vi "WriteResolverParameters.vi"(8 "error in (no error)":errorcluster, 9 "UserValues":dbl[](array[numeric]), 10 "Resolver Parameters in":T1[](array[typedef]), 11 "FPGA Session":u32) -> (0 "error out":errorcluster, 2 "Resolver Parameters out":T1[](array[typedef]), 3 "FPGA Session Out":u32)   [LabVIEW 2011, in "Sensor Simulation Custom Device.lvlib"]
uses:
  Sensor Simulation Custom Device.lvlib
  TypeDefs/Resolver Parameters.ctl
  <userlib>/_FPGA Interface Advanced Tools/FPGA Interface Wrapper/NiFPGA Write - I32.vi
  <vilib>/Utility/error.llb/Error Cluster From Error Code.vi
  <userlib>/_FPGA Interface Advanced Tools/FPGA Interface Wrapper/FPGA Interface Wrapper.lvlib
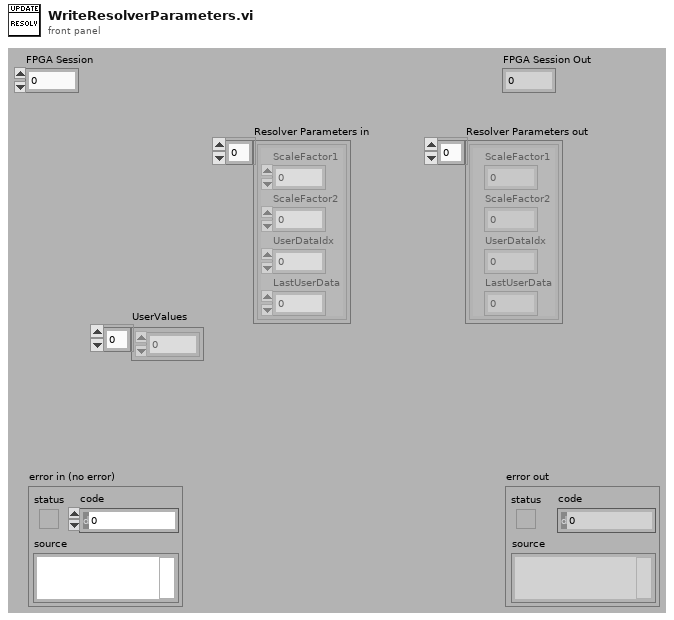
[diagram p1: front panel]
types:
  T1 = typedef "Sensor Simulation Custom Device.lvlib/Resolver Parameters.ctl" = cluster{"ScaleFactor1":u32, "ScaleFactor2":u32, "UserDataIdx":i32, "LastUserData":dbl}
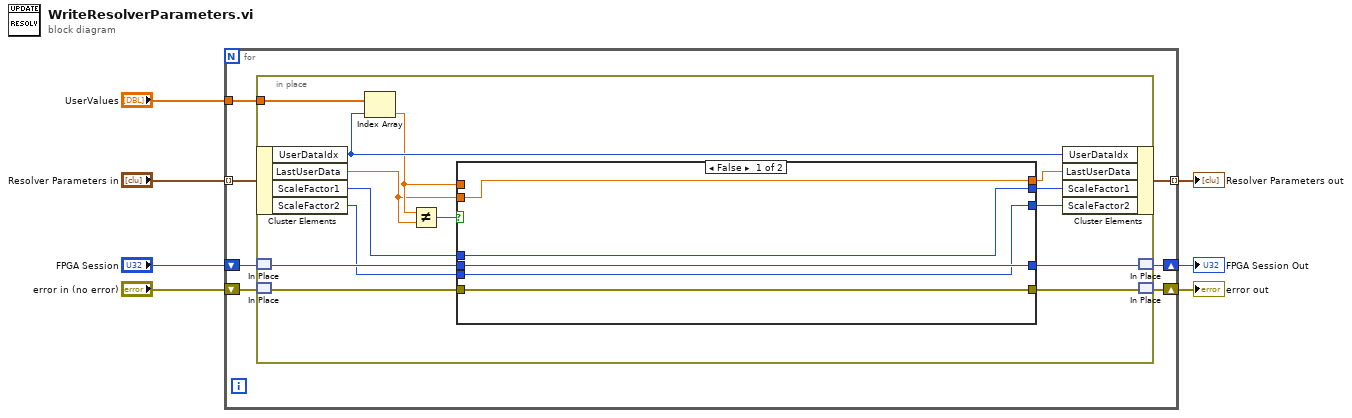
[diagram p0: block diagram]
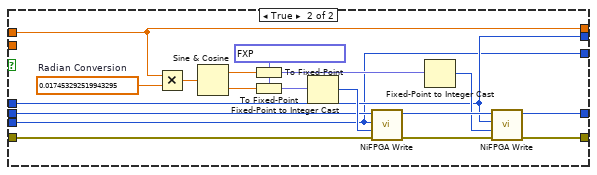
[diagram p2: hidden frame]
diagram:
  n1 = for {
    shift-right: [w11] -> w6
    shift-left: "error in (no error)" -> [w12]
    shift-right: [w10] -> w5
    shift-left: "FPGA Session" -> [w13]
    tunnel: "UserValues" -> [w14]
    tunnel: "Resolver Parameters in" -> [w9] mode=indexing
    tunnel: [w8] -> w1 mode=indexing
    n2 = in-place {
      in-place-border: w14 -> [w28]
      n3 = in-place-cluster #1(w9) -> ("UserDataIdx"=w23:i32, "LastUserData"=w19:dbl, "ScaleFactor1"=w18:u32, "ScaleFactor2"=w17:u32)
      n4 = in-place-match #2(w13) -> (w26:u32)
      n5 = in-place-match #3(w12) -> (w27:errorcluster)
      n6 = Index Array(array=w28, index=w23) -> (element=w21:dbl)
      n7 = Not Equal?(x=w21, y=w19) -> (x != y?=w22:bool)
      n8 = case shown="False" w22 {
        tunnel: w27 -> [w31 w40]
        tunnel: w26 -> [w32 w39]
        tunnel: [w31 w38] -> w25
        tunnel: [w32 w37] -> w24
        tunnel: w21 -> [_ w36]
        tunnel: [w33 w36] -> w20
        tunnel: w19 -> [w33 _]
        tunnel: w17 -> [w30 w34]
        tunnel: w18 -> [w29 w35]
        tunnel: [w30 w34] -> w16
        tunnel: [w29 w35] -> w15
        frame False {
        }
        frame True {
          w45 = 0.017453292519943295  # Radian Conversion
          w47 = fxp<+/-,19,5> 0.0 ("Scaling Factor")
          n9 = Multiply(x=w36, y=w45) -> (x*y=w51:dbl)
          n10 = Sine & Cosine(0:w51) -> (1:w50:dbl, 2:w48:dbl)
          n11 = To Fixed-Point(fixed-point type=w47, number=w50) -> (fixed-point=w49:fxp<+/-,19,5>)
          n12 = To Fixed-Point(fixed-point type=w47, number=w48) -> (fixed-point=w46:fxp<+/-,19,5>)
          n13 = Fixed-Point to Integer Cast(1:w46) -> (0:w44:i32)
          n14 = call-poly <userlib>:"NiFPGA Write.vi"("error in (no error)"=w40, "Value"=w44, "Control"=w34, "Session"=w39) -> ("error out"=w42:errorcluster, "Session Out"=w43:u32)  [unwired: 6 in]
          n15 = Fixed-Point to Integer Cast(1:w49) -> (0:w41:i32)
          n16 = call-poly <userlib>:"NiFPGA Write.vi"("error in (no error)"=w42, "Value"=w41, "Control"=w35, "Session"=w43) -> ("error out"=w38:errorcluster, "Session Out"=w37:u32)  [unwired: 6 in]
        }
      }
      n17 = in-place-cluster #1("UserDataIdx"=w23, "LastUserData"=w20, "ScaleFactor1"=w15, "ScaleFactor2"=w16) -> (w8:T1)
      n18 = in-place-match #2(w24) -> (w10:u32)
      n19 = in-place-match #3(w25) -> (w11:errorcluster)
    }
  }
  "error out" <- w6
  "FPGA Session Out" <- w5
  "Resolver Parameters out" <- w1
